vi "SR_Main.vi"() -> ()   [LabVIEW 2018]
panel:
  out "错误输出":errorcluster
  out "SR_REC_TEXT":string
  in  "停止":bool
  in  "错误输入（无错误）":errorcluster
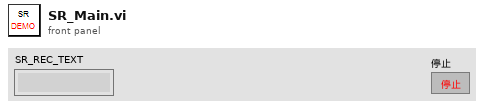
[diagram p1: front panel]
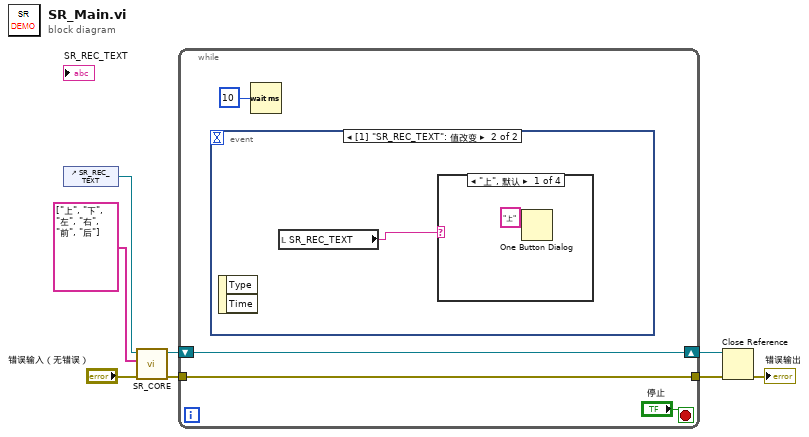
[diagram p0: block diagram]
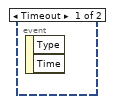
[diagram p2: hidden frame]
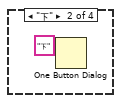
[diagram p3: hidden frame]
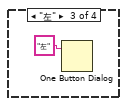
[diagram p4: hidden frame]
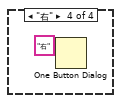
[diagram p5: hidden frame]
diagram:
  n1 = control-ref of="SR_REC_TEXT"() -> (w4:refnum<vi>)
  n2 = call "SR_CORE.vi"("错误输入（无错误）"="错误输入（无错误）", "phrases"=string[] ["上", "下", "左", "右", "前", "后"], "SR_REC_TEXT"=w4) -> ("错误输出"=w3:errorcluster, ".NET引用句柄输出"=w6:refnum<k24>)  [unwired: 7 in]
  n3 = while {
    shift-right: [w10] -> w5
    shift-left: w6 -> [w10]
    tunnel: w3 -> [w9]
    tunnel: [w9] -> w2
    stop <- "停止" stop-if-true
    n4 = event shown="[1] \"SR_REC_TEXT\": 值改变" {
      selector: _ -> [_ _]
      dyn-events: _ -> [_ _]
      timeout: _ -> [_ _]
      event Timeout {
        n5 = event-data() -> ()  [unwired: 1 in, 2 out]
      }
      event "SR_REC_TEXT": Value Change {
        n6 = event-data() -> ()  [unwired: 1 in, 2 out]
        n7 = local read "SR_REC_TEXT"() -> (w13:string)
        n8 = case shown="\"上\", 默认" w13 {
          frame "上", Default {
            n9 = One Button Dialog(message="上") -> ()  [unwired: 2 out]
          }
          frame "下" {
            n10 = One Button Dialog(message="下") -> ()  [unwired: 2 out]
          }
          frame "左" {
            n11 = One Button Dialog(message="左") -> ()  [unwired: 2 out]
          }
          frame "右" {
            n12 = One Button Dialog(message="右") -> ()  [unwired: 2 out]
          }
        }
      }
    }
    n13 = Wait (ms)(milliseconds to wait=u32 10 ("等待时间（毫秒）")) -> ()  [unwired: 1 out]
  }
  n14 = Close Reference(reference=w5, error in (no error)=w2) -> (error out=→"错误输出":errorcluster)
